vi "FPGA Main Image Processing - Single Loop.vi"(9 "?":T1) -> ()   [LabVIEW 2025]
doc: "The myRIO v1.1 FPGA Shipping Personality. This personality contains support for:\n- 2 Analog Input Interrupt channel\n- 4 Digital Input Interrupt channel\n- 1 Timer\n- 1 Accelerometer\n- 1 Button\n- 4 LED\n- 10 Analog Input channels with 1 Sample\n- 6 Analog Output channels with 1 Sample\n- 40 Digital I/O channels with 1 Sample\n- 2 I2C channels\n- 4 Encoder channels\n- 6 PWM channels\n- 2 SPI channels"
uses:
  SoC IP Library/Controls/Ocurrences.ctl
  SoC IP Library/Controls/Image Size.ctl
  <vilib>/rvi/Emulation/niFpgaGetClockAttributes.vi
  <vilib>/rvi/Emulation/niFpgaSctlEmulationGetInTimedLoop.vi
  <vilib>/rvi/Emulation/niFpgaEmulationReportErrorSimple.vi
  <vilib>/eio/utilities/niEioResolveVilibRelativePath.vi
  <vilib>/rvi/interface/RandomDataEmulation/niFpgaRandomDataHandleErrors.vi
  <vilib>/rvi/Memory/Memory_Emulation/nirvimemoryFastEmulation.vi
  <vilib>/rvi/Memory/Memory_Emulation/nirvimemoryEmulation.vi
  <vilib>/rvi/Emulation/niFpgaEmulationIsFPGAContextNoSignature.vi
  <vilib>/rvi/DataTransferAndStorage/Container/Common/niFpgaContainerGetUniqueNameForEmu.vi
  <vilib>/rvi/Emulation/niFpgaProcessEmulError.vi
  <vilib>/rvi/errors/nirviReportUnexpectedCaseInternalError (U32).vi
  <vilib>/rvi/Emulation/niFpgaCriticalErrorInLSC.vi
  <vilib>/rvi/DataTransferAndStorage/Container/Common/niFpgaContainerSetEmuInfo.vi
  <vilib>/rvi/eio/common/nirviEmuReportErrorAndStop.vi
  <vilib>/rvi/DataTransferAndStorage/Container/Common/niFpgaContainerExecOnDevCompGetState.vi
  <vilib>/rvi/Memory/Memory_Emulation/niFpgaMemoryEmulationCacheClearOnFirstRun.vi
  <vilib>/rvi/Memory/Memory_Emulation/nirvimemoryEmulationManagerCache_MakeExclusive.vi
  <vilib>/rvi/Memory/Memory_Emulation/niFpgaMemoryEmulationValidateCache.vi
  <vilib>/rvi/Memory/Memory_Emulation/nirvimemoryEmulationManagerCache_InsertValue.vi
  <vilib>/Utility/error.llb/Clear Errors.vi
  <vilib>/rvi/Memory/Memory_Emulation/nirvimemoryEmulationManagerCache_ReleaseExclusive.vi
  <vilib>/rvi/Memory/Memory_Emulation/nirvimemoryEmulationManagerCache_GetValue.vi
  <vilib>/rvi/Memory/Memory_Emulation/nirvimemoryEmulationManagerCache_SetValue.vi
  <vilib>/rvi/Emulation/niFpgaSctlEmulationResourceMgr.vi
  <vilib>/rvi/DataTransferAndStorage/Container/XNode/niFpgaContainer.xnode
  <vilib>/rvi/interface/RandomDataEmulation/nirviRandomDataFpgaReadWriteTemplate.vi
  <vilib>/rvi/LocalResourceManager/LocalResourceManager.xnode
  <vilib>/rvi/Memory/Memory_Emulation/niFpgaMemoryEmulationRefIn.vi
  SoC IP Library/SoC IP Library.lvlib
panel:
  out "Write TO":bool
  out "Read TO":bool
  out "Pixel B Write":u32
  out "Pixel A Write":u32
  out "Last Processed Pixel?":bool
  out "Pixel":u32
  out "Processing iteration":i32=-1
  out "Current Colum Process":u32
  out "Current Row Process":u32
  out "Current Colum Write":u32
  out "Current Row Write":u32
  out "Last Write Pixel?":bool
  out "Last Read Pixel?":bool
  out "Current Colum Read":u32
  out "Current Row Read":u32
  out "Pixel B Write":u32
  out "Pixel A Write":u32
  out "Pixel B Read":u32
  out "Pixel A Read":u32
  out "SYS.OCURRENCES.RDY":bool
  out "FPGA to RT iteration":i32=-1
  out "RT to FPGA iteration":i32=-1
  out "SYS.IMG_SIZE.RDY":bool
  out "Image size":u32
  out "SYS.RDY":bool
  # "Image Processing"
  # "System"
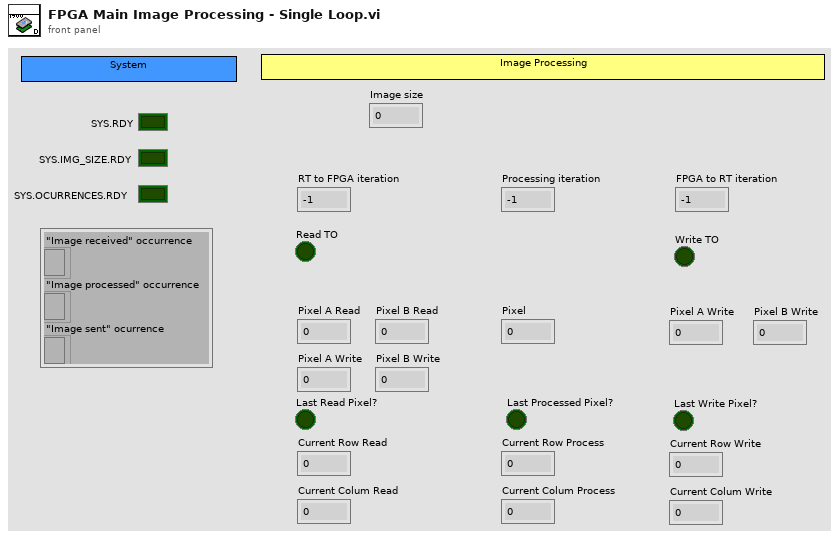
[diagram p1: front panel]
types:
  T1 = typedef "SoC IP Library.lvlib/Ocurrences.ctl" = cluster{"\"Image received\" occurrence":refnum<k4>, "\"Image processed\" occurrence":refnum<k4>, "\"Image sent\" ocurrence":refnum<k4>}
  T2 = typedef "SoC IP Library.lvlib/Image Size.ctl" = cluster{"Rows (X)":u16, "Colums (Y)":u16}
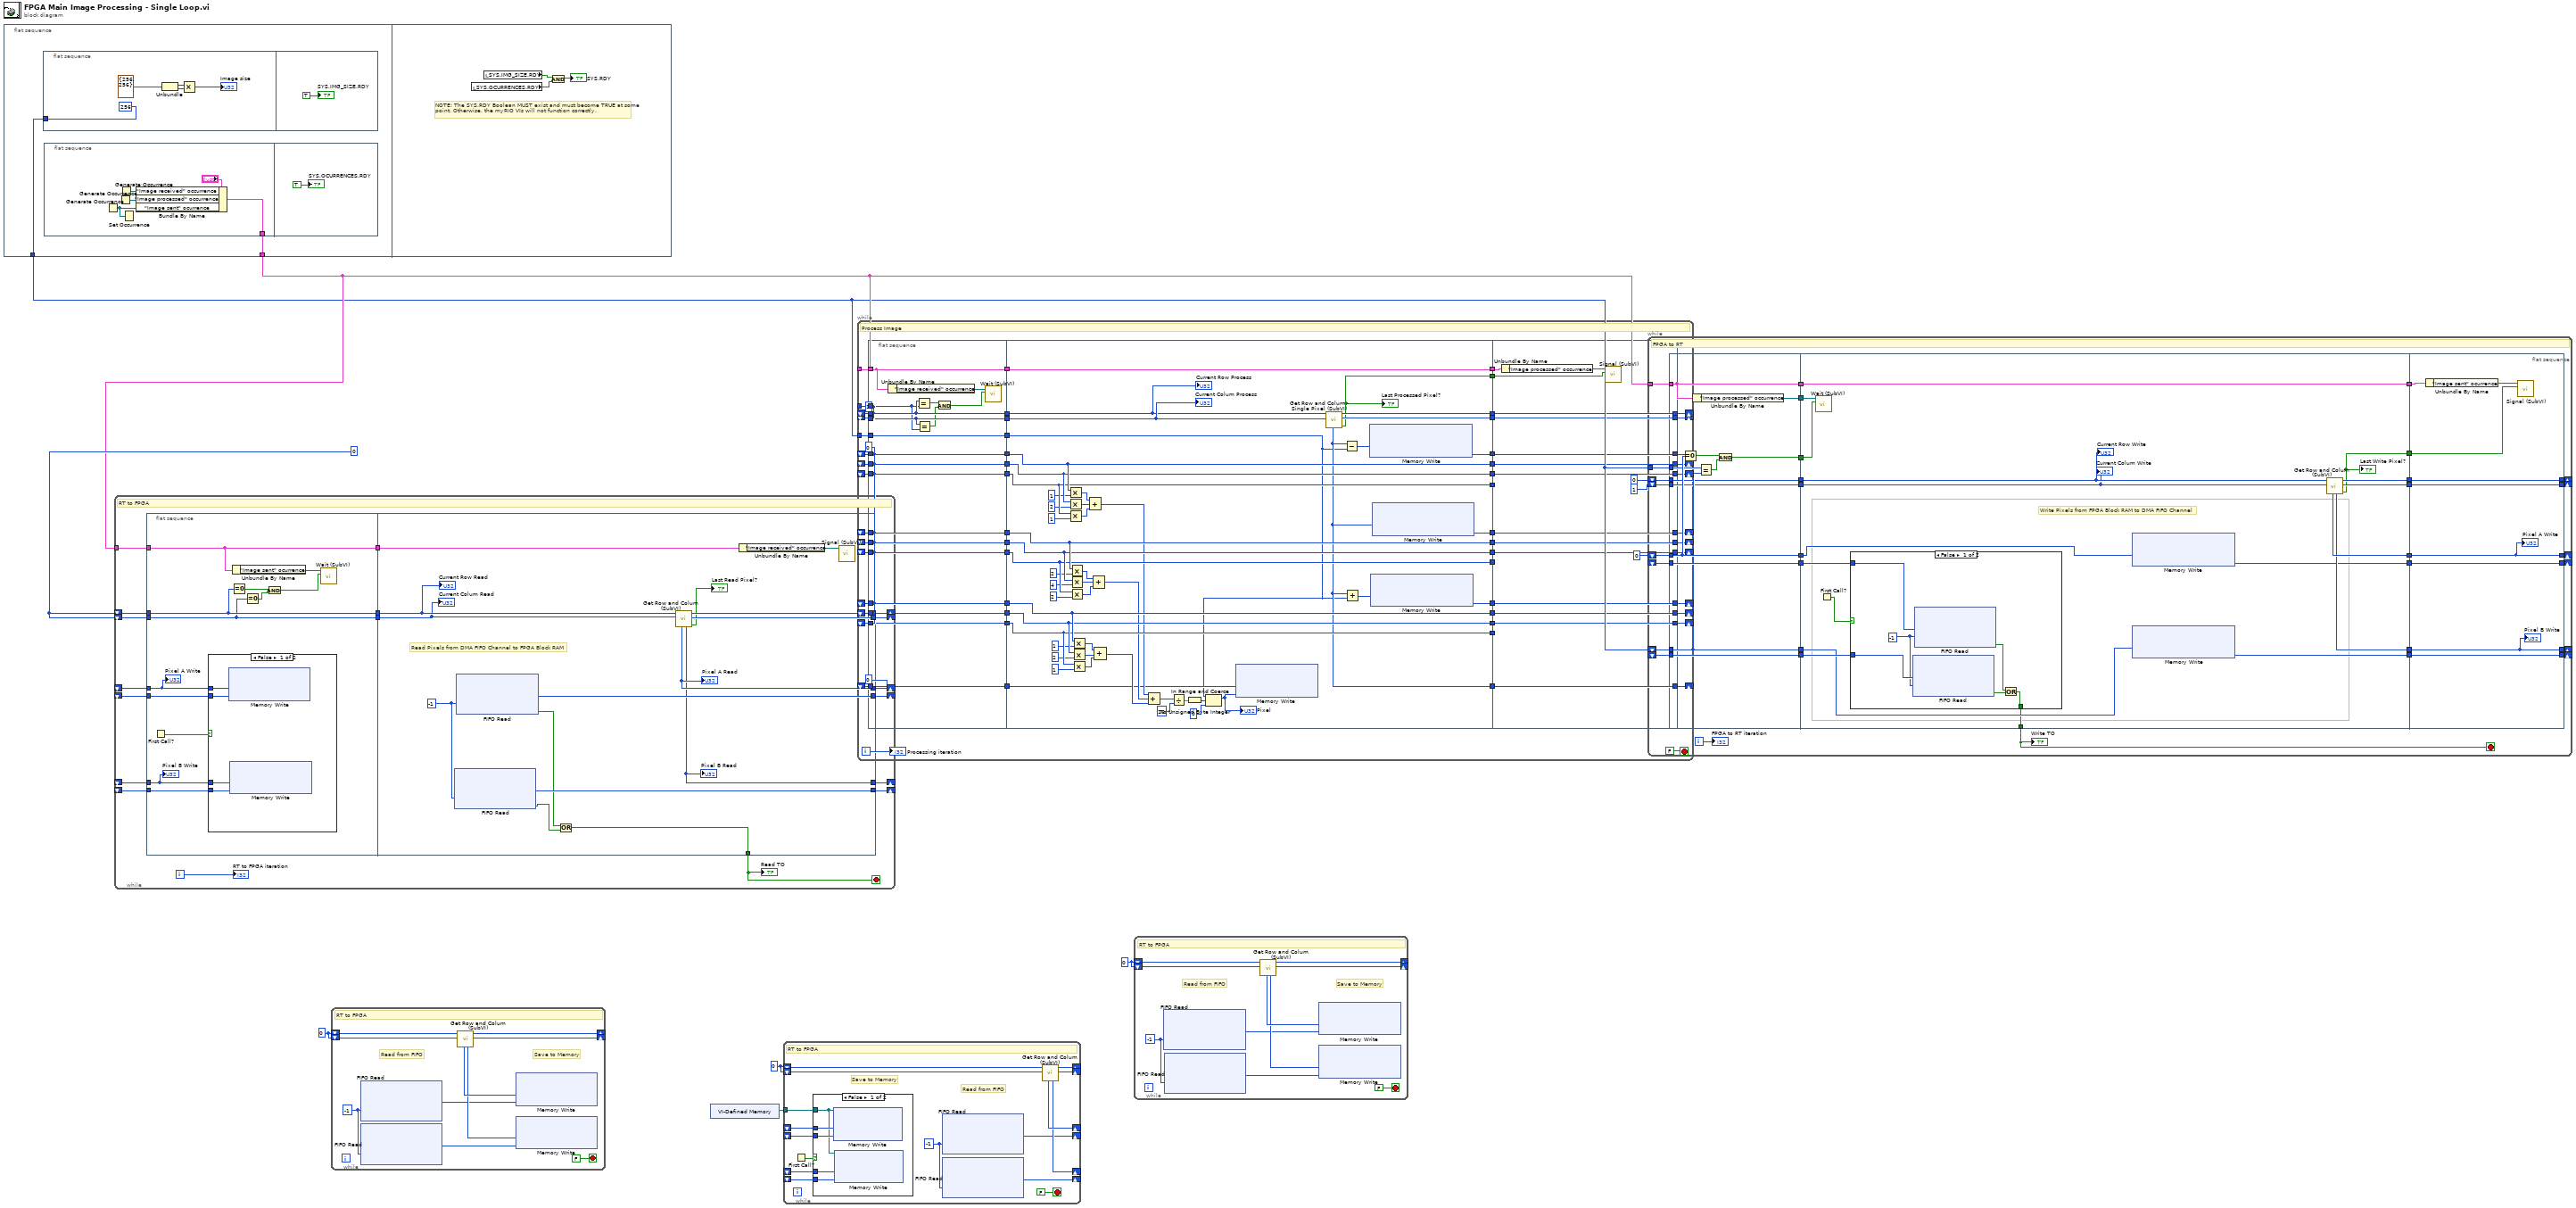
[diagram p0: block diagram]
diagram:
  w2 = u8 0
  w3 = u8 0
  w4 = u8 0
  w5 = u8 0 ("Data")
  w6 = u32 1 ("Row Out")
  w11 = u32 0
  n1 = flat-sequence {
    tunnel: [w15] -> w8
    tunnel: [w14] -> w9
    frame #0 {
      n2 = flat-sequence {
        tunnel: [u32 256 ("Dimension")] -> w15
        frame #0 {
          n3 = Unbundle(T2 {"Rows (X)"=256, "Colums (Y)"=256} ("Image Size")) -> ("Rows (X)"=w24:u16, "Colums (Y)"=w25:u16)
          n4 = Multiply(x=w24, y=w25) -> (x*y=→"Image size":u32)
        }
        frame #1 {
          "SYS.IMG_SIZE.RDY" <- TRUE
        }
      }
      n5 = flat-sequence {
        tunnel: [w16] -> w14
        frame #0 {
          n6 = Generate Occurrence() -> (w17:refnum<k4>)
          n7 = Generate Occurrence() -> (w18:refnum<k4>)
          n8 = Generate Occurrence() -> (w19:refnum<k4>)
          n9 = Set Occurrence(w17) -> ()
          n10 = Bundle By Name(cluster="?", "\"Image received\" occurrence"=w19, "\"Image processed\" occurrence"=w18, "\"Image sent\" ocurrence"=w17) -> (w16:T1)
        }
        frame #1 {
          "SYS.OCURRENCES.RDY" <- TRUE
        }
      }
    }
    frame #1 {
      # "NOTE: The SYS.RDY Boolean MUST exist and must become TRUE at some point. Otherwise, the myRIO VIs will not function correctly."
      n11 = local read "SYS.OCURRENCES.RDY"() -> (w29:bool)
      n12 = local read "SYS.IMG_SIZE.RDY"() -> (w28:bool)
      n13 = And(x=w28, y=w29) -> (x .and. y?=→"SYS.RDY":bool)
    }
  }
  n14 = while {
    shift-right: [w40] -> _
    shift-left: _ -> [w47]
    shift-right: [w34] -> _
    shift-left: _ -> [w46]
    shift-right: [w39] -> _
    shift-left: _ -> [w45]
    shift-right: [w43] -> _
    shift-left: _ -> [w44]
    shift-right: [w42] -> _
    shift-left: w11 -> [w38]
    shift-right: [w41] -> _
    shift-left: w11 -> [w37]
    tunnel: w9 -> [w33]
    i -> [w48]
    stop <- w31 stop-if-true
    # "RT to FPGA"
    n15 = flat-sequence {
      tunnel: w37 -> [w58]
      tunnel: w38 -> [w59]
      tunnel: w44 -> [w52]
      tunnel: w45 -> [w50]
      tunnel: w46 -> [w53]
      tunnel: w47 -> [w51]
      tunnel: [w59] -> w36
      tunnel: [w58] -> w35
      tunnel: w33 -> [w60]
      tunnel: [w60] -> w32
      tunnel: w36 -> [w75]
      tunnel: w35 -> [w74]
      tunnel: w32 -> [w72]
      tunnel: [w79] -> w34
      tunnel: [w78] -> w43
      tunnel: [w77] -> w42
      tunnel: [w76] -> w41
      tunnel: [w71] -> w40
      tunnel: [w70] -> w39
      tunnel: [w66] -> w31
      frame #0 {
        n16 = First Call?() -> (First Call?: T/F=w54:bool)
        n17 = case shown="False" w54 {
          tunnel: w51 -> [w64 _]
          tunnel: w53 -> [w62 _]
          tunnel: w52 -> [w61 _]
          tunnel: w50 -> [w63 _]
          frame False {
            n18 = xnode ("Memory Write")("Address"=w64, "Data"=w62) -> ()  [unwired: 1 in, 1 out]
            n19 = xnode ("Memory Write")("Address"=w63, "Data"=w61) -> ()  [unwired: 1 in, 1 out]
          }
          frame True {
          }
        }
        n20 = Equal To 0?(x=w59) -> (x = 0?=w57:bool)
        n21 = Unbundle By Name(w60) -> ("\"Image sent\" ocurrence"=w56:refnum<k4>)
        n22 = Equal To 0?(x=w58) -> (x = 0?=w55:bool)
        n23 = And(x=w57, y=w55) -> (x .and. y?=w49:bool)
        n24 = call "Wait (SubVI).vi"("Wait? (T)"=w49, "Occurrence in"=w56) -> ()  [unwired: 10 in]
        "Pixel A Write" <- w51
        "Pixel B Write" <- w50
      }
      frame #1 {
        w65 = -1 ("Timeout")
        # "Read Pixels from DMA FIFO Channel to FPGA Block RAM"
        n25 = xnode ("FIFO Read")("Timeout"=w65) -> ("Element"=w78:u8, "Timed Out?"=w67:bool)  [unwired: 1 in, 1 out]
        n26 = xnode ("FIFO Read")("Timeout"=w65) -> ("Element"=w79:u8, "Timed Out?"=w68:bool)  [unwired: 1 in, 1 out]
        n27 = Or(x=w68, y=w67) -> (x .or. y?=w66:bool)
        n28 = call "Get Row and Colum (SubVI).vi"("Colum In"=w74, "Row In"=w75) -> ("Last Pixel?"=→"Last Read Pixel?":bool, "Colum Out"=w76:u8, "Row Out"=w77:u8, "Pixel B"=w70:u16, "Pixel A"=w71:u16)  [unwired: 5 in]
        "Pixel A Read" <- w71
        "Pixel B Read" <- w70
        n29 = Unbundle By Name(w72) -> ("\"Image received\" occurrence"=w69:refnum<k4>)
        n30 = call "Signal (SubVI).vi"("Occurrence in"=w69) -> ()  [unwired: 11 in]
        "Current Row Read" <- w75
        "Current Colum Read" <- w74
      }
    }
    "RT to FPGA iteration" <- w48
    "Read TO" <- w31
  }
  n31 = while {
    shift-right: [w89] -> _
    shift-left: w4 -> [w87]
    shift-right: [w88] -> _
    shift-left: w4 -> [w86]
    stop <- FALSE stop-if-true
    w84 = -1 ("Timeout")
    # "Save to Memory"
    # "Read from FIFO"
    # "RT to FPGA"
    n32 = xnode ("FIFO Read")("Timeout"=w84) -> ("Element"=w81:u8)  [unwired: 1 in, 2 out]
    n33 = xnode ("FIFO Read")("Timeout"=w84) -> ("Element"=w80:u8)  [unwired: 1 in, 2 out]
    n34 = call "Get Row and Colum (SubVI).vi"("Colum In"=w86, "Row In"=w87) -> ("Colum Out"=w88:u8, "Row Out"=w89:u8, "Pixel B"=w82:u16, "Pixel A"=w83:u16)  [unwired: 5 in, 1 out]
    n35 = xnode ("Memory Write")("Address"=w83, "Data"=w81) -> ()  [unwired: 1 in, 1 out]
    n36 = xnode ("Memory Write")("Address"=w82, "Data"=w80) -> ()  [unwired: 1 in, 1 out]
  }
  n37 = xnode "VI-Defined Memory"() -> ("Memory Out"=w1:refnum<k21>)
  n38 = while {
    shift-right: [w98] -> _
    shift-left: _ -> [w105]
    shift-right: [w94] -> _
    shift-left: _ -> [w104]
    shift-right: [w97] -> _
    shift-left: _ -> [w103]
    shift-right: [w101] -> _
    shift-left: _ -> [w102]
    shift-right: [w100] -> _
    shift-left: w3 -> [w96]
    shift-right: [w99] -> _
    shift-left: w3 -> [w95]
    tunnel: w1 -> [w90]
    stop <- FALSE stop-if-true
    w91 = -1 ("Timeout")
    # "Read from FIFO"
    # "Save to Memory"
    # "RT to FPGA"
    n39 = First Call?() -> (First Call?: T/F=w92:bool)
    n40 = case shown="False" w92 {
      tunnel: w105 -> [w110 _]
      tunnel: w104 -> [w108 _]
      tunnel: w102 -> [w107 _]
      tunnel: w103 -> [w109 _]
      tunnel: w90 -> [w106 _]
      frame False {
        n41 = xnode ("Memory Write")("Address"=w110, "Data"=w108, "Memory In"=w106) -> ()  [unwired: 1 out]
        n42 = xnode ("Memory Write")("Address"=w109, "Data"=w107, "Memory In"=w106) -> ()  [unwired: 1 out]
      }
      frame True {
      }
    }
    n43 = xnode ("FIFO Read")("Timeout"=w91) -> ("Element"=w94:u8)  [unwired: 1 in, 2 out]
    n44 = xnode ("FIFO Read")("Timeout"=w91) -> ("Element"=w101:u8)  [unwired: 1 in, 2 out]
    n45 = call "Get Row and Colum (SubVI).vi"("Colum In"=w95, "Row In"=w96) -> ("Colum Out"=w99:u8, "Row Out"=w100:u8, "Pixel B"=w97:u16, "Pixel A"=w98:u16)  [unwired: 5 in, 1 out]
  }
  n46 = while {
    tunnel: w9 -> [w169]
    shift-right: [w165] -> _
    shift-left: w5 -> [w163]
    shift-right: [w161] -> _
    shift-left: w5 -> [w160]
    shift-right: [w157] -> _
    shift-left: w5 -> [w155]
    shift-right: [w152] -> _
    shift-left: w5 -> [w150]
    shift-right: [w148] -> _
    shift-left: w5 -> [w146]
    shift-right: [w144] -> _
    shift-left: w5 -> [w142]
    shift-right: [w139] -> _
    shift-left: w5 -> [w138]
    shift-right: [w135] -> _
    shift-left: w5 -> [w134]
    shift-right: [w131] -> _
    shift-left: w5 -> [w129]
    shift-right: [w126] -> _
    shift-left: w6 -> [w121]
    shift-right: [w124] -> _
    shift-left: w6 -> [w122]
    tunnel: w8 -> [w119]
    shift-right: [w115] -> _
    shift-left: u32 0 ("Pixel") -> [w117]
    tunnel: w6 -> [w113]
    i -> [w111]
    stop <- FALSE stop-if-true
    # "Process Image"
    n47 = flat-sequence {
      tunnel: w169 -> [w188]
      tunnel: [w188] -> w167
      tunnel: [w187] -> w164
      tunnel: w163 -> [w187]
      tunnel: w160 -> [w186]
      tunnel: [w186] -> w159
      tunnel: [w185] -> w156
      tunnel: w155 -> [w185]
      tunnel: [w184] -> w151
      tunnel: w150 -> [w184]
      tunnel: [w183] -> w147
      tunnel: w146 -> [w183]
      tunnel: [w182] -> w143
      tunnel: w142 -> [w182]
      tunnel: w138 -> [w181]
      tunnel: [w181] -> w137
      tunnel: w134 -> [w180]
      tunnel: [w180] -> w133
      tunnel: [w179] -> w130
      tunnel: w129 -> [w179]
      tunnel: [w176] -> w123
      tunnel: w122 -> [w176]
      tunnel: w121 -> [w175]
      tunnel: [w175] -> w120
      tunnel: w119 -> [w178]
      tunnel: [w178] -> w118
      tunnel: w117 -> [w177]
      tunnel: [w177] -> w116
      tunnel: w113 -> [w174]
      tunnel: [w239] -> w168
      tunnel: w167 -> [w239]
      tunnel: [w238] -> w166
      tunnel: w164 -> [w235]
      tunnel: [w235] -> w162
      tunnel: w159 -> [w234]
      tunnel: [w234] -> w158
      tunnel: w156 -> [w233]
      tunnel: [w233] -> w154
      tunnel: [w237] -> w153
      tunnel: w151 -> [w232]
      tunnel: [w232] -> w149
      tunnel: w147 -> [w231]
      tunnel: [w231] -> w145
      tunnel: w143 -> [w230]
      tunnel: [w230] -> w141
      tunnel: [w236] -> w140
      tunnel: w137 -> [w229]
      tunnel: [w229] -> w136
      tunnel: w133 -> [w228]
      tunnel: [w228] -> w132
      tunnel: w130 -> [w227]
      tunnel: [w227] -> w128
      tunnel: [w205] -> w127
      tunnel: [w204] -> w125
      tunnel: w123 -> [w195]
      tunnel: w120 -> [w196]
      tunnel: w118 -> [w197]
      tunnel: w116 -> [w201]
      tunnel: [w200] -> w114
      tunnel: [w194] -> w112
      tunnel: w168 -> [w254]
      tunnel: w166 -> [w252]
      tunnel: [w252] -> w165
      tunnel: w162 -> [w251]
      tunnel: [w251] -> w161
      tunnel: w158 -> [w250]
      tunnel: [w250] -> w157
      tunnel: w154 -> [_]
      tunnel: w153 -> [w249]
      tunnel: [w249] -> w152
      tunnel: w149 -> [w248]
      tunnel: [w248] -> w148
      tunnel: w145 -> [w247]
      tunnel: [w247] -> w144
      tunnel: w141 -> [_]
      tunnel: w140 -> [w246]
      tunnel: [w246] -> w139
      tunnel: w136 -> [w245]
      tunnel: [w245] -> w135
      tunnel: w132 -> [w244]
      tunnel: [w244] -> w131
      tunnel: w128 -> [_]
      tunnel: [w243] -> w126
      tunnel: w127 -> [w243]
      tunnel: w125 -> [w242]
      tunnel: [w242] -> w124
      tunnel: [w241] -> w115
      tunnel: w114 -> [w241]
      tunnel: w112 -> [w240]
      frame #0 {
        n48 = Unbundle By Name(w188) -> ("\"Image received\" occurrence"=w189:refnum<k4>)
        n49 = Equal?(x=w176, y=w174) -> (x = y?=w173:bool)
        n50 = Equal?(x=w175, y=w174) -> (x = y?=w172:bool)
        n51 = And(x=w173, y=w172) -> (x .and. y?=w171:bool)
        n52 = call "Wait (SubVI).vi"("Wait? (T)"=w171, "Occurrence in"=w189) -> ()  [unwired: 10 in]
      }
      frame #1 {
        n53 = Multiply(x=w235, y=i16 1) -> (x*y=w221:i16)
        n54 = Multiply(x=w234, y=i16 2) -> (x*y=w223:i16)
        n55 = Multiply(x=w233, y=i16 1) -> (x*y=w222:i16)
        n56 = Multiply(x=w232, y=i16 2) -> (x*y=w220:i16)
        n57 = Multiply(x=w231, y=i16 4) -> (x*y=w219:i16)
        n58 = Multiply(x=w230, y=i16 2) -> (x*y=w218:i16)
        n59 = Multiply(x=w229, y=i16 1) -> (x*y=w226:i16)
        n60 = Multiply(x=w228, y=i16 2) -> (x*y=w225:i16)
        n61 = Multiply(x=w227, y=i16 1) -> (x*y=w224:i16)
        n62 = Compound Arithmetic op=ADD(w221, w223, w222) -> (w217:i16)
        n63 = Compound Arithmetic op=ADD(w220, w219, w218) -> (w216:i16)
        n64 = Compound Arithmetic op=ADD(w226, w225, w224) -> (w215:i16)
        n65 = Compound Arithmetic op=ADD(w217, w216, w215) -> (w193:i16)
        n66 = Divide(x=w193, y=i16 16) -> (x/y=w191:fxp<+,8,8>)
        n67 = To Unsigned Byte Integer(number=w191) -> (unsigned 8bit integer=w190:u8)
        n68 = In Range and Coerce(upper limit=w197, x=w190, lower limit=i16 0) -> (coerced(x)=w199:u32)  [unwired: 1 out]
        "Pixel" <- w199
        n69 = xnode ("Memory Write")("Address"=w201, "Data"=w199) -> ()  [unwired: 1 in, 1 out]
        n70 = call "Get Row and Colum - Single Pixel (SubVI).vi"("Colum In"=w196, "Row In"=w195) -> ("Last Pixel?"=w194:bool, "Colum Out"=w205:u8, "Row Out"=w204:u8, "Pixel"=w200:u16)  [unwired: 6 in]
        "Last Processed Pixel?" <- w194
        n71 = Subtract(x=w200, y=w197) -> (x-y=w202:u32)
        n72 = Add(x=w200, y=w197) -> (x+y=w203:u32)
        n73 = xnode ("Memory Write")("Address"=w202) -> ("Data"=w238:u8)  [unwired: 1 in, 1 out]
        n74 = xnode ("Memory Write")("Address"=w203) -> ("Data"=w236:u8)  [unwired: 1 in, 1 out]
        n75 = xnode ("Memory Write")("Address"=w200) -> ("Data"=w237:u8)  [unwired: 1 in, 1 out]
        "Current Row Process" <- w195
        "Current Colum Process" <- w196
      }
      frame #2 {
        n76 = Unbundle By Name(w254) -> ("\"Image processed\" occurrence"=w253:refnum<k4>)
        n77 = call "Signal (SubVI).vi"("Set? (T)"=w240, "Occurrence in"=w253) -> ()  [unwired: 10 in]
      }
    }
    "Processing iteration" <- w111
  }
  n78 = while {
    shift-right: [w264] -> _
    shift-left: w2 -> [w262]
    shift-right: [w263] -> _
    shift-left: w2 -> [w261]
    stop <- FALSE stop-if-true
    w259 = -1 ("Timeout")
    # "Save to Memory"
    # "Read from FIFO"
    # "RT to FPGA"
    n79 = xnode ("FIFO Read")("Timeout"=w259) -> ("Element"=w256:u8)  [unwired: 1 in, 2 out]
    n80 = xnode ("FIFO Read")("Timeout"=w259) -> ("Element"=w255:u8)  [unwired: 1 in, 2 out]
    n81 = call "Get Row and Colum (SubVI).vi"("Colum In"=w261, "Row In"=w262) -> ("Colum Out"=w263:u8, "Row Out"=w264:u8, "Pixel B"=w257:u16, "Pixel A"=w258:u16)  [unwired: 5 in, 1 out]
    n82 = xnode ("Memory Write")("Address"=w258, "Data"=w256) -> ()  [unwired: 1 in, 1 out]
    n83 = xnode ("Memory Write")("Address"=w257, "Data"=w255) -> ()  [unwired: 1 in, 1 out]
  }
  n84 = while {
    shift-right: [w293] -> _
    shift-left: u32 0 -> [w297]
    shift-right: [w292] -> _
    shift-left: w8 -> [w296]
    shift-right: [w295] -> _
    shift-left: u32 0 -> [w291]
    shift-right: [w294] -> _
    shift-left: u32 1 ("Colum Out") -> [w290]
    shift-right: [w280] -> _
    shift-left: _ -> [w276]
    shift-right: [w278] -> _
    shift-left: _ -> [w274]
    tunnel: w8 -> [w270]
    tunnel: w9 -> [w269]
    i -> [w282]
    stop <- w265 stop-if-true
    # "FPGA to RT"
    n85 = flat-sequence {
      tunnel: w290 -> [w301]
      tunnel: w291 -> [w302]
      tunnel: w296 -> [w304]
      tunnel: w297 -> [w305]
      tunnel: [w305] -> w289
      tunnel: [w304] -> w288
      tunnel: [w307] -> w277
      tunnel: w276 -> [w307]
      tunnel: [w306] -> w275
      tunnel: w274 -> [w306]
      tunnel: [w303] -> w273
      tunnel: [w302] -> w272
      tunnel: [w301] -> w271
      tunnel: w270 -> [w300]
      tunnel: w269 -> [w299]
      tunnel: [w299] -> w268
      tunnel: [w298] -> w266
      tunnel: w289 -> [w317]
      tunnel: w288 -> [w316]
      tunnel: [w327] -> w287
      tunnel: [w326] -> w286
      tunnel: [w325] -> w285
      tunnel: [w324] -> w284
      tunnel: [w323] -> w283
      tunnel: [w322] -> w281
      tunnel: [w321] -> w279
      tunnel: w277 -> [w320]
      tunnel: w275 -> [w319]
      tunnel: w273 -> [w310]
      tunnel: w272 -> [w315]
      tunnel: w271 -> [w314]
      tunnel: w268 -> [w313]
      tunnel: [w313] -> w267
      tunnel: w266 -> [w312]
      tunnel: [w311] -> w265
      tunnel: [w339] -> w292
      tunnel: [w340] -> w293
      tunnel: [w341] -> w294
      tunnel: [w342] -> w295
      tunnel: w287 -> [w342]
      tunnel: w286 -> [w341]
      tunnel: w285 -> [w340]
      tunnel: w284 -> [w339]
      tunnel: w283 -> [w334]
      tunnel: [w338] -> w280
      tunnel: w281 -> [w338]
      tunnel: [w337] -> w278
      tunnel: w279 -> [w337]
      tunnel: w267 -> [w336]
      frame #0 {
        n86 = Equal To 0?(x=w305) -> (x = 0?=w308:bool)
        n87 = Unbundle By Name(w299) -> ("\"Image processed\" occurrence"=w298:refnum<k4>)
        n88 = Equal?(x=w300, y=w304) -> (x = y?=w309:bool)
        n89 = And(x=w308, y=w309) -> (x .and. y?=w303:bool)
      }
      frame #1 {
        # "Write Pixels from FPGA Block RAM to DMA FIFO Channel"
        n90 = call "Wait (SubVI).vi"("Wait? (T)"=w310, "Occurrence in"=w312) -> ()  [unwired: 10 in]
        n91 = First Call?() -> (First Call?: T/F=w318:bool)
        n92 = case shown="False" w318 {
          tunnel: w320 -> [w333 _]
          tunnel: w319 -> [w332 _]
          tunnel: [w329 _] -> w311
          frame False {
            w328 = -1 ("Timeout")
            n93 = xnode ("FIFO Read")("Element"=w332, "Timeout"=w328) -> ("Timed Out?"=w331:bool)  [unwired: 1 in, 1 out]
            n94 = xnode ("FIFO Read")("Element"=w333, "Timeout"=w328) -> ("Timed Out?"=w330:bool)  [unwired: 1 in, 1 out]
            n95 = Or(x=w330, y=w331) -> (x .or. y?=w329:bool)
          }
          frame True {
          }
        }
        n96 = xnode ("Memory Write")("Address"=w317) -> ("Data"=w322:u8)  [unwired: 1 in, 1 out]
        n97 = xnode ("Memory Write")("Address"=w316) -> ("Data"=w321:u8)  [unwired: 1 in, 1 out]
        n98 = call "Get Row and Colum (SubVI).vi"("Colum In"=w314, "Row In"=w315) -> ("Last Pixel?"=w323:bool, "Colum Out"=w326:u8, "Row Out"=w327:u8, "Pixel B"=w324:u16, "Pixel A"=w325:u16)  [unwired: 5 in]
        "Last Write Pixel?" <- w323
        "Current Row Write" <- w315
        "Current Colum Write" <- w314
      }
      frame #2 {
        n99 = Unbundle By Name(w336) -> ("\"Image sent\" ocurrence"=w335:refnum<k4>)
        n100 = call "Signal (SubVI).vi"("Set? (T)"=w334, "Occurrence in"=w335) -> ()  [unwired: 10 in]
        "Pixel A Write" <- w340
        "Pixel B Write" <- w339
      }
    }
    "FPGA to RT iteration" <- w282
    "Write TO" <- w265
  }
